vi "ep_Transpose 3D Array.vi"(11 "Array":dbl[][][](array[numeric])) -> (3 "Array out":dbl[][][](array[numeric]))   [LabVIEW 2012]
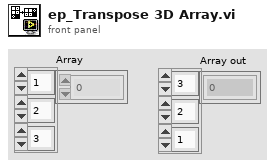
[diagram p1: front panel]
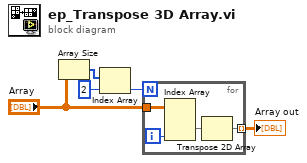
[diagram p0: block diagram]
diagram:
  n1 = Array Size(array="Array") -> (size(s)=w5:i32[])
  n2 = Index Array(array=w5, index=2) -> (element=w4:i32)
  n3 = for {
    N: w4 -> [_]
    tunnel: "Array" -> [w9]
    tunnel: [w6] -> w2 mode=indexing
    i -> [w8]
    n4 = Index Array(array=w9, index (dim 2)=w8) -> (element=w7:dbl[][])  [unwired: 2 in]
    n5 = Transpose 2D Array(2D array=w7) -> (transposed array=w6:dbl[][])
  }
  "Array out" <- w2
